vi "Draw.vi"(8 "error in (no error)":errorcluster, 10 "picture in (empty picture)":picture, 11 "Line in":refnum<class "Line.lvclass">) -> (0 "error out":errorcluster, 2 "picture out":picture, 3 "Line out":refnum<class "Line.lvclass">)   [LabVIEW 2018, in "Line.lvclass"]
doc: "Draw a line"
uses:
  Line.lvclass
  Graphics Object/Graphics Object.lvclass
panel:
  # "expressionflow.com"
  # "Copyright (c) 2008 Tomi Maila. All rights reserved."
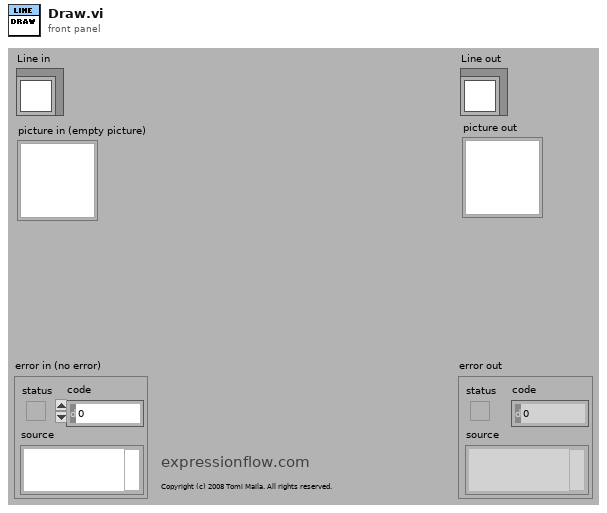
[diagram p1: front panel]
types:
  T1 = cluster{"Width":u16, "Style":enum32{"Solid", "Dash", "Dot", "DashDot", "DashDotDot"}}
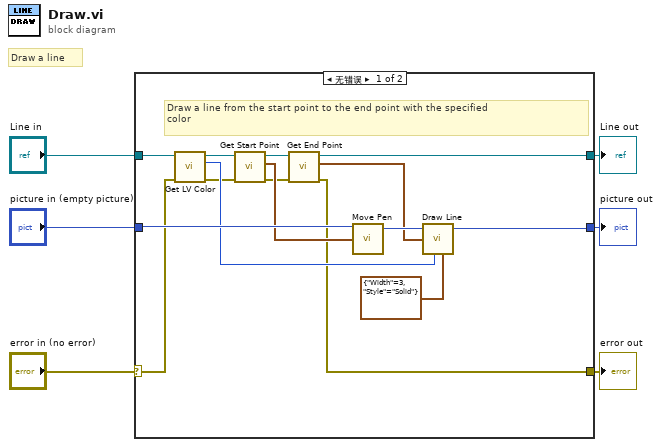
[diagram p0: block diagram]
diagram:
  # "Draw a line"
  n1 = case shown="无错误" "error in (no error)" {
    selector: "error in (no error)" -> [w16 w23]
    tunnel: [w18 w24] -> w5
    tunnel: "picture in (empty picture)" -> [w21 w24]
    tunnel: [w7 w23] -> w3
    tunnel: [w11 w22] -> w2
    tunnel: "Line in" -> [w17 w22]
    frame No Error {
      # "Draw a line from the start point to the end point with the specified \ncolor"
      n2 = call-dynamic "Get LV Color.vi"("error in (no error)"=w16, "Graphics Object.lvclass in"=w17) -> ("error out"=w8:errorcluster, "Color"=w19:u32, "Graphics Object.lvclass out"=w14:refnum<class "Line.lvclass">)  [unwired: 7 in]
      n3 = call "Get Start Point.vi"("error in (no error)"=w8, "Graphics Object.lvclass in"=w14) -> ("error out"=w9:errorcluster, "start point"=w13:cluster{"x":i16, "y":i16}, "Graphics Object.lvclass out"=w12:refnum<class "Line.lvclass">)  [unwired: 7 in]
      n4 = call "Get End Point.vi"("error in (no error)"=w9, "Graphics Object.lvclass in"=w12) -> ("error out"=w7:errorcluster, "end point"=w10:cluster{"x":i16, "y":i16}, "Graphics Object.lvclass out"=w11:refnum<class "Line.lvclass">)  [unwired: 7 in]
      n5 = call <vilib>:"Move Pen.vi"("new position"=w13, "picture"=w21) -> ("new picture"=w20:picture)  [unwired: 3 in]
      n6 = call <vilib>:"Draw Line.vi"("picture"=w20, "end point"=w10, "color(black)"=w19, "pen"=T1 {"Width"=3, "Style"=enum."Solid"}) -> ("new picture"=w18:picture)  [unwired: 5 in]
    }
    frame Error {
    }
  }
  "error out" <- w3
  "Line out" <- w2
  "picture out" <- w5
